vi "RMAD logger.vi"() -> ()   [LabVIEW 2017]
panel:
  out "regobs from inifile":T1(array[cluster]) {"regobs_ObsLocation" items=["Ikke gitt"=0, "Lauvjuvet"=66553, "Sandneslia"=66555, "Lauvjuvet Demo"=47721, "Sandneslia Demo"=47724, "Lauvjuvet Test"=62943, "Sandneslia Test"=62942, "F46 test"=63942, "F46 Demo"=47760]; "regobs_AvalancheTriggerTID" items=["Ikke gitt"=0, "Naturlig utløst"=10, "Kunstig utløst"=20, "Ski eller skuter utløst"=21, "Ski eller skuter fjernutløst"=22, "Kunstig utløst testheng"=23, "Utløst med sprengstoff"=25, "Ukjent"=99]; "regobs_AvalancheTID" items=["Ikke gitt"=0, "Tørt løssnøskred"=12, "Vått løssnøskred"=11, "Tørt flakskred"=22, "Vått flakskred"=21, "Glideskred"=27, "Sørpeskred"=30, "Skavlfall"=40, "Ukjent"=99]; "regobs_TerrainStartZoneTID" items=["Ikke gitt"=0, "Brattheng"=10, "Leområder"=20, "Nær rygg"=30, "I renne eller forsenkning"=40, "Svaberg"=50, "Skål"=60, "I skogen"=70, "Hogstfelt"=75, "Overalt i terrenget"=95, "Ukjent"=99]}
  out "Trafikkontroll terskelverdier":T2(array[cluster])
  out "Stredstørrelser terskelverdier":T3(array[cluster])
  in  "Tab Control":T4(tab)
  out "Skredhendelser":T5(array[cluster]) {"Intensitet terskel 1" format="%.1f"; "Intensitet terskel 2" format="%.1f"; "Intensitet terskel 3" format="%.1f"; "Intensitet terskel 4" format="%.1f"; "Intensitet terskel 5" format="%.1f"}
  out "is logging":bool[](array[boolean])
  out "registration in regObs":T6(array[cluster]) {"DestructiveSizeTID" items=["Ikke gitt"=0, "1-Harmløs"=1, "2-Små"=2, "3-Middels"=3, "4-Stort"=4, "5-Svært stort"=5, "Ukjent"=9]; "TerrainStartZoneTID" items=["Ikke gitt"=0, "Brattheng"=10, "Leområder"=20, "Nær rygg"=30, "I renne eller forsenkning"=40, "Svaberg"=50, "Skål"=60, "I skogen"=70, "Hogstfelt"=75, "Overalt i terrenget"=95, "Ukjent"=99]; "AvalancheTID" items=["Ikke gitt"=0, "Tørt løssnøskred"=12, "Vått løssnøskred"=11, "Tørt flakskred"=22, "Vått flakskred"=21, "Glideskred"=27, "Sørpeskred"=30, "Skavlfall"=40, "Ukjent"=99]; "AvalancheTriggerTID" items=["Ikke gitt"=0, "Naturlig utløst"=10, "Kunstig utløst"=20, "Ski eller skuter utløst"=21, "Ski eller skuter fjernutløst"=22, "Kunstig utløst testheng"=23, "Utløst med sprengstoff"=25, "Ukjent"=99]}
  out "registration ID":string[](array[string])
  in  "?":T7(tab)
  out "Nedlastede data 1":waveform(dbl)[](graph)
  out "Nedlastede data 2":waveform(dbl)[](graph)
  out "Nedlastede data 3":waveform(dbl)[](graph)
  out "Nedlastede data 4":waveform(dbl)[](graph)
  out "Nedlastede data 5":waveform(dbl)[](graph)
  in  "Download dataset":bool
  in  "Node":i32=1
  in  "ID":u16
  in  "Start Logging":bool
  out "Recent events":T8(array[cluster]) {"SPS" format="%.1f"}
  out "Temperatur":waveform(dbl)[](graph)
  out "Batteri spenning":waveform(dbl)[](graph)
  out "Radio Latency":waveform(i32)[](graph)
  out "Avalanch Packets":T9(array[cluster]) {"A1 std" format="%.1f"; "A2 std" format="%.1f"; "A3 std" format="%.1f"; "A4 std" format="%.1f"; "A1 ratio" format="%.1g"; "A2 ratio" format="%.1g"; "A3 ratio" format="%.1g"; "A4 ratio" format="%.1g"}
  out "Avalanch JBV":T10(array[cluster]) {"A2 mean" format="%.1f"; "A1 mean" format="%.1f"; "A1 std" format="%.1f"; "A2 std" format="%.1f"}
  in  "Send Reset":bool
  in  "SetAUX":bool
  in  "Node":u8=1
  in  "Get Status":bool
  in  "AUX min int":u16=15
  out "AUX data":T11(array[cluster]) {"Node configuration"."configuration" items=[""=100, "Radio Repeater"=0, "Geofon"=1, "Sensornode"=2, "Jernbane"=3, "Infralyd"=4]; "Node configuration"."radio config" items=[""=100, "Smartmesh IP"=0]; "batteri (V)" format="%.3g"; "temperatur (c)" format="%.1g"; "?" format="%#.5g"}
  out "Mote Status":T12(array[cluster]) {"mote state" items=["Lost"=0, "Negotiating"=1, "Operational"=4]}
  out "Link status":T13(array[cluster])
  out "Safe download":T14(array[cluster])
  out "NGI Packets Dust":cluster{"MAc Adress":string, "data":string}[](array[cluster])
  out "dust manager mac adress":string
  out "mac adress":string[](array[string])
  out "radio IO":errorcluster
  in  "stop":bool
  out "gateway IP":T15={"serial_mux IP"="127.0.0.1", "serial_mux port"=9900}
  out "event_datadir":string
  out "aux_datadir":string
  out "mesh_datadir":string
  out "sec since last packet":dbl
  out "Gateway Info":T16
  out "Gateway Status":T17
  out "node names":string[](array[string])
  in  "max download atempts":u8=3
  out "auto_download_enabled":bool
  out "gateway_snmp_enabled":bool
  out "RMAD signalys monitor enabled":bool
  out "vdv_datadir":string
  out "ini file":path
  out "regObs baseurl":string
  out "RMAD Signalys Monitor":T18 {"Uptime  (W:D:H)" format="%<%W:%D:%H>t"}
  out "error regObs":errorcluster
  out "error signalys":errorcluster
  out "error snmp":errorcluster
  in  "download timeout":dbl=180.0 format="%#_13g"
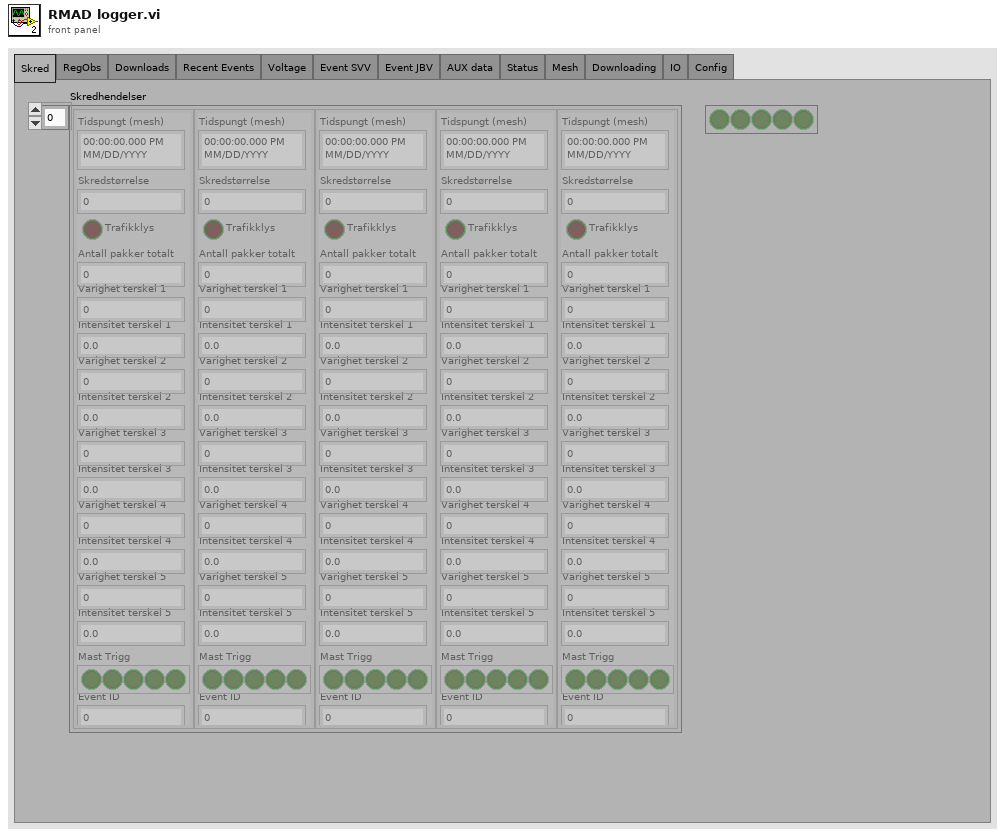
[diagram p1: front panel]
types:
  T1 = cluster{"regobs_ObsLocation":i32, "regobs_AvalancheTriggerTID":i32, "regobs_AvalancheTID":i32, "regobs_TerrainStartZoneTID":i32, "regobs_Trajectory":string, "regobs_ValidExposition":string, "regobs_startLat":dbl, "regobs_startLong":dbl, "regobs_stopLat":dbl[], "regobs_stopLong":dbl[], "regobs_heading":u32, "regobs_velocity":u32, "regobs_comment":string}[]
  T2 = cluster{"terskelverdi":u32, "antall sensorer":u32, "varighet":u32}[]
  T3 = cluster{"teskelverdi":u32, "antall sensorer":u32, "varighet":u32}[][]
  T4 = enum32{"Skred", "RegObs", "Downloads", "Recent Events", "Voltage", "Event SVV", "Event JBV", "AUX data", "Status", "Mesh", "Downloading", "IO", "Config"}
  T5 = cluster{"Tidspungt (mesh)":timestamp, "Skredstørrelse":i32, "Trafikklys":bool, "Antall pakker totalt":u16, "Varighet terskel 1":u16, "Intensitet terskel 1":dbl, "Varighet terskel 2":u16, "Intensitet terskel 2":dbl, "Varighet terskel 3":u16, "Intensitet terskel 3":dbl, "Varighet terskel 4":u16, "Intensitet terskel 4":dbl, "Varighet terskel 5":u16, "Intensitet terskel 5":dbl, "Mast Trigg":bool[], "Event ID":i32}[]
  T6 = cluster{"DtAvalancheTime (UTC)":string, "DestructiveSizeTID":i32, "AvalancheTriggerTID":i32, "AvalancheTID":i32, "TerrainStartZoneTID":i32, "ValidExposition":string, "Trajectory":string, "StartLat":dbl, "StartLong":dbl, "StopLat":dbl, "StopLong":dbl, "Comment":string}[]
  T7 = enum32{"Mast 1", "Mast 2", "Mast 3", "Mast 4", "Mast 5"}
  T8 = cluster{"ID":u16, "Timestamp":timestamp, "Packets":u16, "SPS":dbl, "Samples":u16}[][]
  T9 = cluster{"time (mesh)":timestamp, "Limit reached flagg":bool[], "A1 std":sgl, "A2 std":sgl, "A3 std":sgl, "A4 std":sgl, "A1 ratio":sgl, "A2 ratio":sgl, "A3 ratio":sgl, "A4 ratio":sgl, "A1 max":u16, "A2 max":u16, "A3 max":u16, "A4 max":u16, "A1 min":u16, "A2 min":u16, "A3 min":u16, "A4 min":u16, "A1 maxS":u16, "A2 maxS":u16, "A3 maxS":u16, "A4 maxS":u16, "A1 minS":u16, "A2 minS":u16, "A3 minS":u16, "A4 minS":u16}[]
  T10 = cluster{"Dust Timestamp":timestamp, "Limit reached flagg":bool[], "A1 std":sgl, "A2 std":sgl, "A1 mean":sgl, "A2 mean":sgl, "A1 max":i32, "A2 max":i32, "A1 min":i32, "A2 min":i32, "A1 maxS":u16, "A2 maxS":u16, "A1 minS":u16, "A2 minS":u16}[]
  T11 = cluster{"Node configuration":cluster{"configuration":u8, "sw vertion":u8, "hw revition":u8, "radio config":u8}, "flaggs":bool[], "batteri (V)":dbl, "temperatur (c)":dbl, "is singed int?":bool[], dbl[], "last update (pc time)":timestamp}[]
  T12 = cluster{"mac adress":string, "mote state":u8, "temperature (C)":i8, "battery (mV)":u16, "avg latecy":u32, "requested bw":u32, "good neighbour":u8, "num neighbour":u8, "num lost packets":u8, "last update (pc)":timestamp}[]
  T13 = cluster{"source mac adress":string, cluster{"destination":string, "rssi":i8, "TxPackets":u16}[], "last update":timestamp}[]
  T14 = cluster{"this instance":bool, "download ID":u32, "samples in dataset":u32, "num  samples":u32, "downloading":bool, "complete":bool, "attempts":u32, "timeout clock":timestamp}[]
  T15 = cluster{"serial_mux IP":string, "serial_mux port":u16}
  T16 = cluster{"Name":string, "Location":string, "Gateway":string, "Firmware":string, "Serial Number":string}
  T17 = cluster{"Supply Voltage":dbl, "Temperatur":u32, "DI":bool, "DO":bool}
  T18 = cluster{"Uptime  (W:D:H)":dbl, "status error":bool, "output enabled":bool, "Last update":timestamp}
  T19 = enum16{"big-endian, network order", "native, host order", "little-endian"}
  T20 = cluster{"Device Health Report":cluster{"MAC adress":string, "charge (mC)":u32, "queueOcc":u8, "temperature (C)":i8, "batteryVoltage (mV)":u16, "numTxOk":u16, "numTxFail":u16, "numRxOK":u16, "numRxFail":u16, "numMACdropped":u8, "numTxBad":u8, "badLinkFrameID":u8, "badLinkSlot":u32, "badLinkOffset":u8}, "mote staus event":cluster{"data":string, u8}, "getMoteInfo":cluster{"MAC adress":string, "state":u8, "numNbrs":u8, "numGoodNbrs":u8, "requestedBw":u32, "totalNeededBw":u32, "assignedBw":u32, "packetsRecived":u32, "packetsLost":u32, "avgLatecy":u32}, "GetPathInfo":cluster{"Path ID":u8, "Src MAC":string, "Dest MAC":string, "direction":u8, "numLinks":u8, "quality":u8, "rssiScrDest":i8, "rssiDestScr":i8}, "Neighbors Health Report":cluster{"MAC adress":string, "neighbourHRdata":cluster{"neighbourID":u16, "neighborFlag":u8, "rssi":i8, "numTxPackets":u16, "numTxFailures":u16, "numRxPackets":u16}[]}, "Discovered Nighbors Health Report":cluster{"MAC adress":string, "numJoinParents":u8, cluster{"neighborID":u16, "rssi":i8, "numRx":u8}[]}, "Mote Config":cluster{"mac adress":string, "MoteID":u16, "isAP":bool, "mote state":u8, "reserved":u8, "isRouting":bool}}
  T21 = cluster{"MAc Adress":string, "UTC Time":timestamp, "srcPort":u16, "dstPort":u16, "data":string}
  T22 = cluster{"Is logging":bool, "num avalanch":u16, "logging startet":timestamp}[]
  T23 = cluster{"ID":u16, "CH mask":u8, "First scan":u32, "Last scans":u32, "Samples":i32[][]}[]
  T24 = cluster{"Dust Timestamp":timestamp, "Limit reached flagg":bool[], "A1 std":sgl, "A2 std":sgl, "A3 std":sgl, "A4 std":sgl, "A1 rat":sgl, "A2 rat":sgl, "A3 rat":sgl, "A4 rat":sgl, "A1 max":u16, "A2 max":u16, "A3 max":u16, "A4 max":u16, "A1 min":u16, "A2 min":u16, "A3 min":u16, "A4 min":u16, "A1 maxS":u16, "A2 maxS":u16, "A3 maxS":u16, "A4 maxS":u16, "A1 minS":u16, "A2 minS":u16, "A3 minS":u16, "A4 minS":u16}[]
  T25 = cluster{"Tidspungt (mesh)":timestamp, "Skredstørrelse":u16, "Trafikklys":bool, "Antall pakker totalt":u16, "Varighet terskel 1":u16, "Intensitet terskel 1":dbl, "Varighet terskel 2":u16, "Intensitet terskel 2":dbl, "Varighet terskel 3":u16, "Intensitet terskel 3":dbl, "Varighet terskel 4":u16, "Intensitet terskel 4":dbl, "Varighet terskel 5":u16, "Intensitet terskel 5":dbl, "Mast Trigg":bool[], "Event ID":i32}[]
  T26 = cluster{"DtAvalancheTime":string, "DestructiveSizeTID":i32, "AvalancheTriggerTID":i32, "AvalancheTID":i32, "TerrainStartZoneTID":i32, "ValidExposition":string, "Trajectory":string, "StartLat":dbl, "StartLong":dbl, "StopLat":dbl, "StopLong":dbl, "Comment":string}[]
  T27 = cluster{"this instance":bool, "download ID":u32, "samples in dataset":u32, "num downloaded samples":u32, "is downloading":bool, "dataset complete":bool, "download attempts":u32, "timeout clock":timestamp}[]
  T28 = cluster{"Mote Temperature":waveform(i32)[], "Mote Battery":waveform(i32)[], "Mote Average Latency":waveform(i32)[]}
  T29 = cluster{"source mac adress":string, cluster{"destination mac":string, "rssi":i8, "numTxPackets":u16}[], "last update":timestamp}[]
  T30 = typedef "LVDateTimeRec.ctl" = cluster{"fractional second":dbl, "second":i32, "minute":i32, "hour":i32, "day of month":i32, "month":i32, "year":i32, "day of week":i32, "day of year":i32, "DST":i32}
  T31 = cluster{"serial_mux IP":string, "rserial_mux port":u16}
  T32 = cluster{"dust master mac":string, "xbee master mac":string, "master name":string, "dust mac":string[], "xbee mac":string[], "node names":string[]}
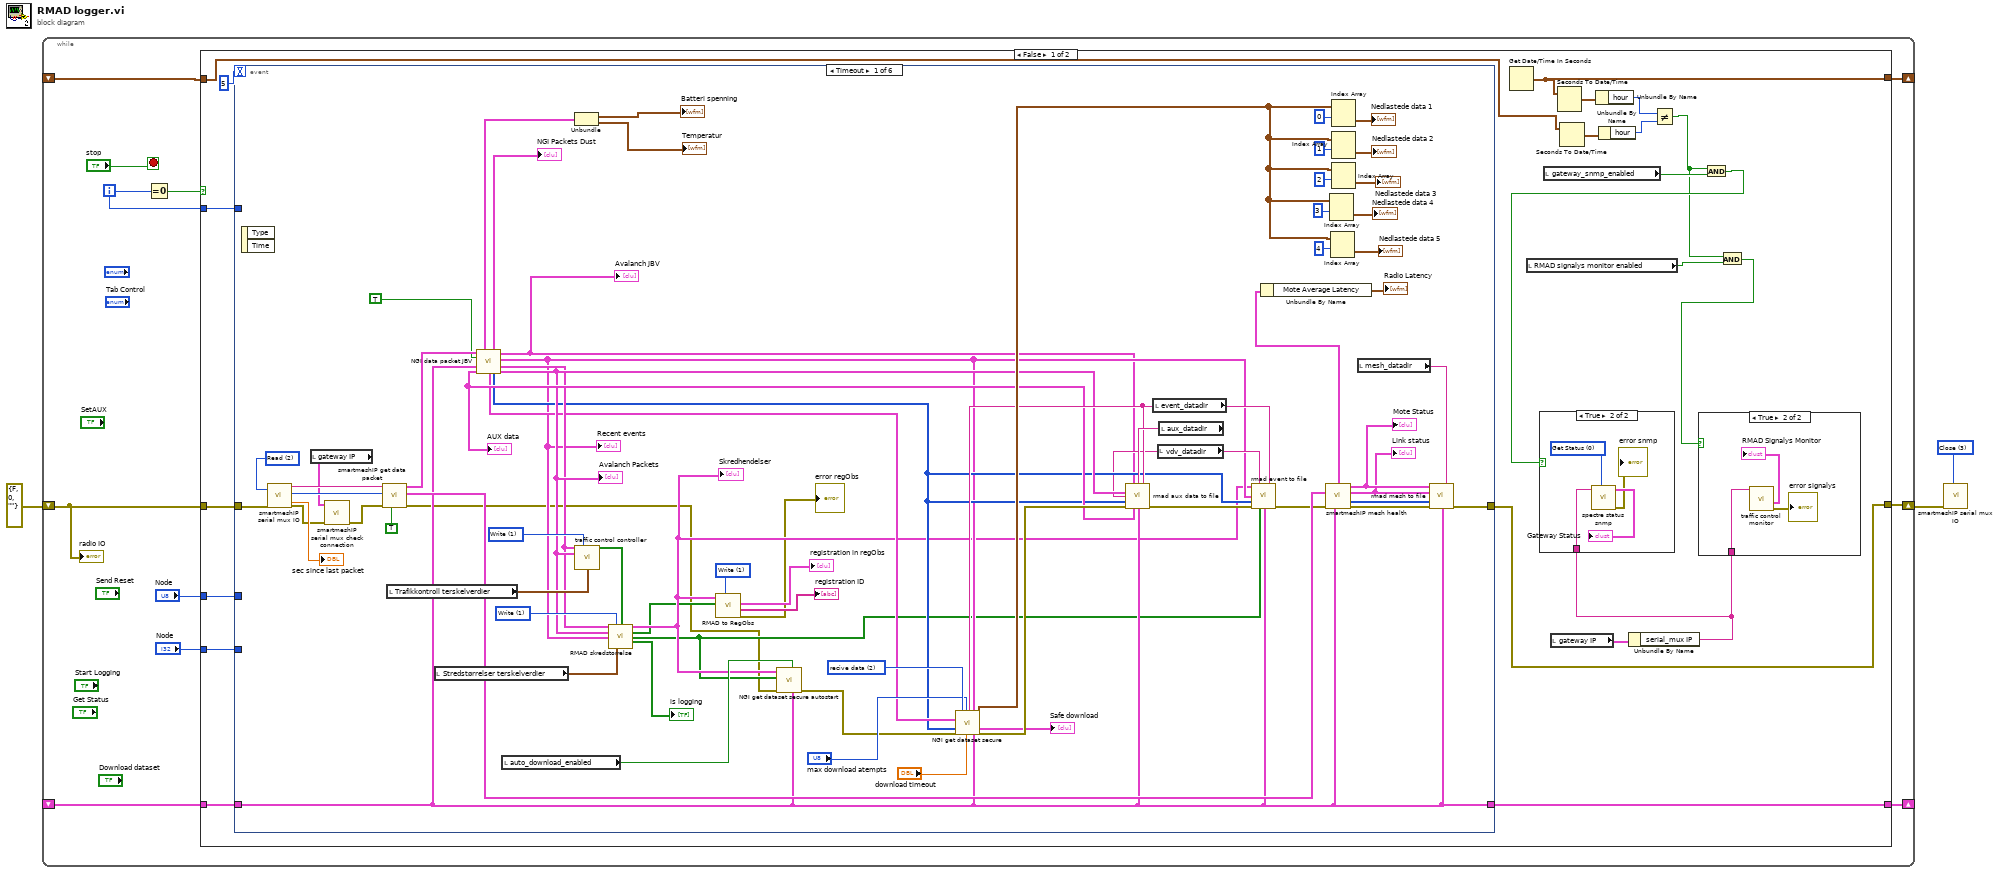
[diagram p0: block diagram]
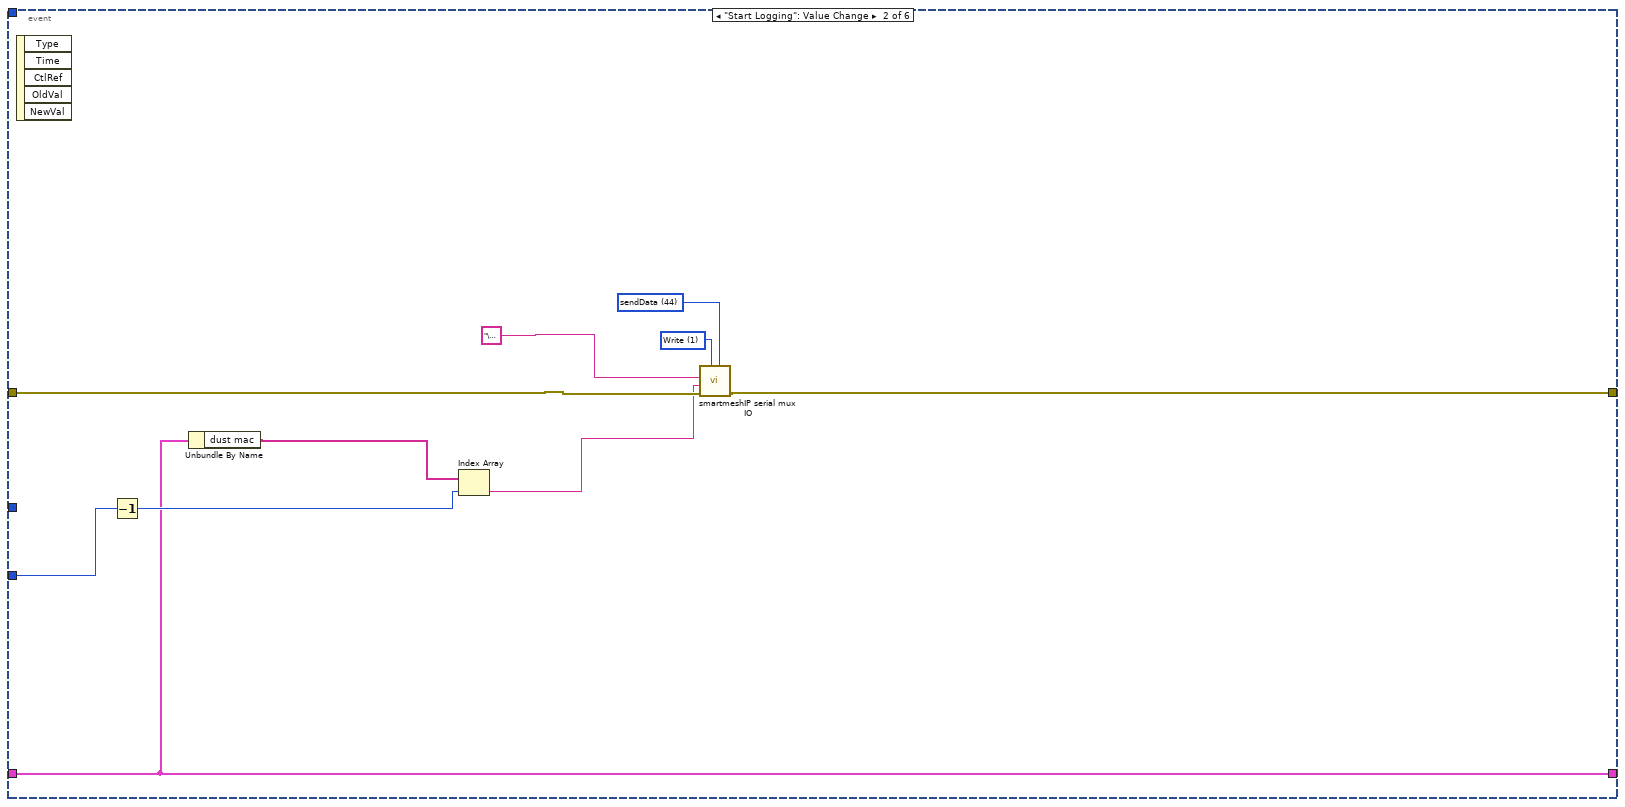
[diagram p4: hidden frame]
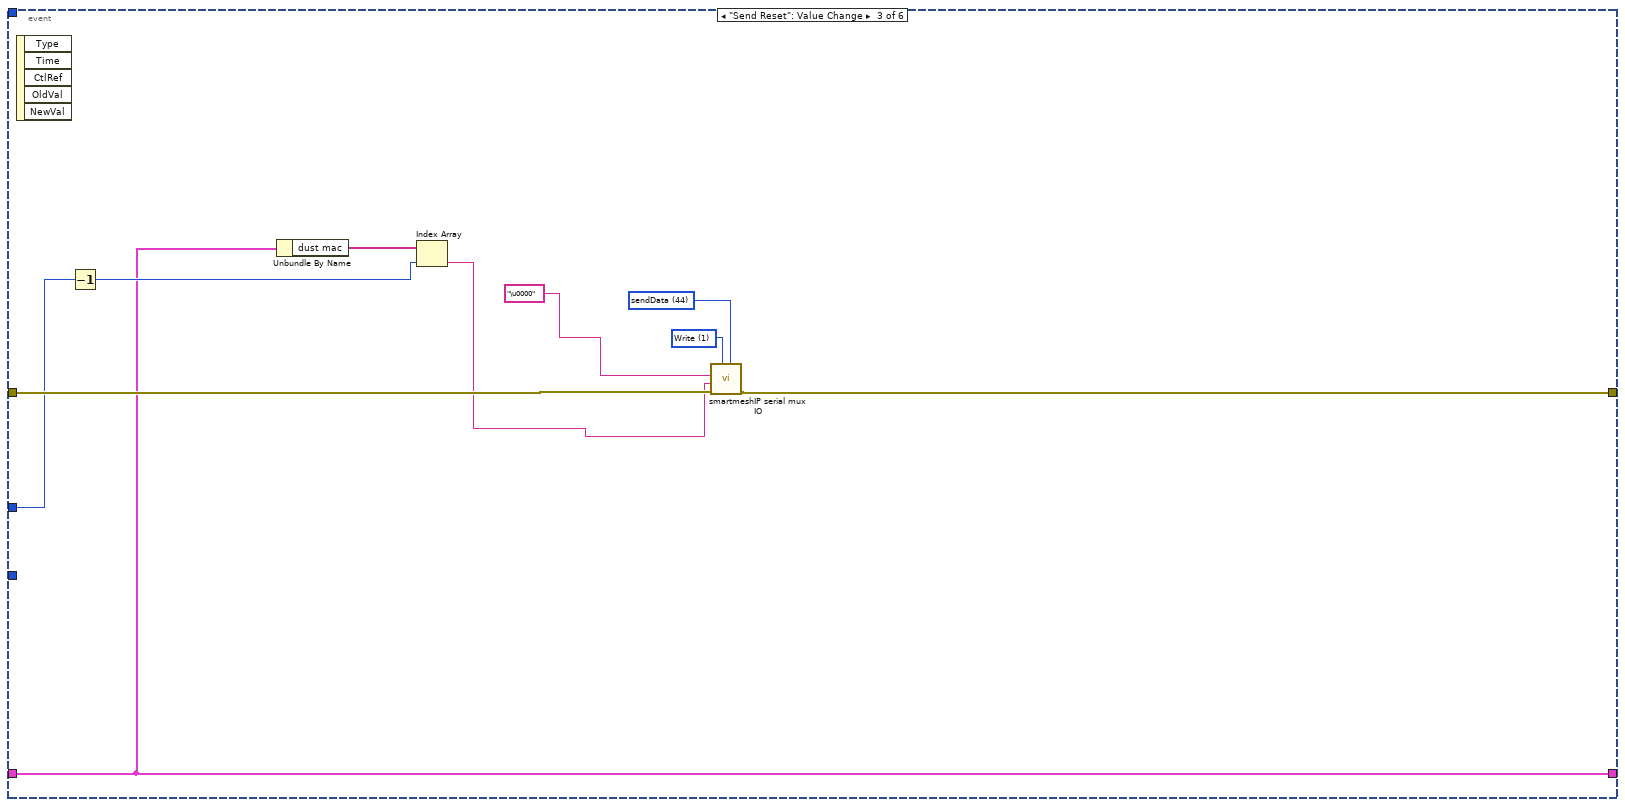
[diagram p5: hidden frame]
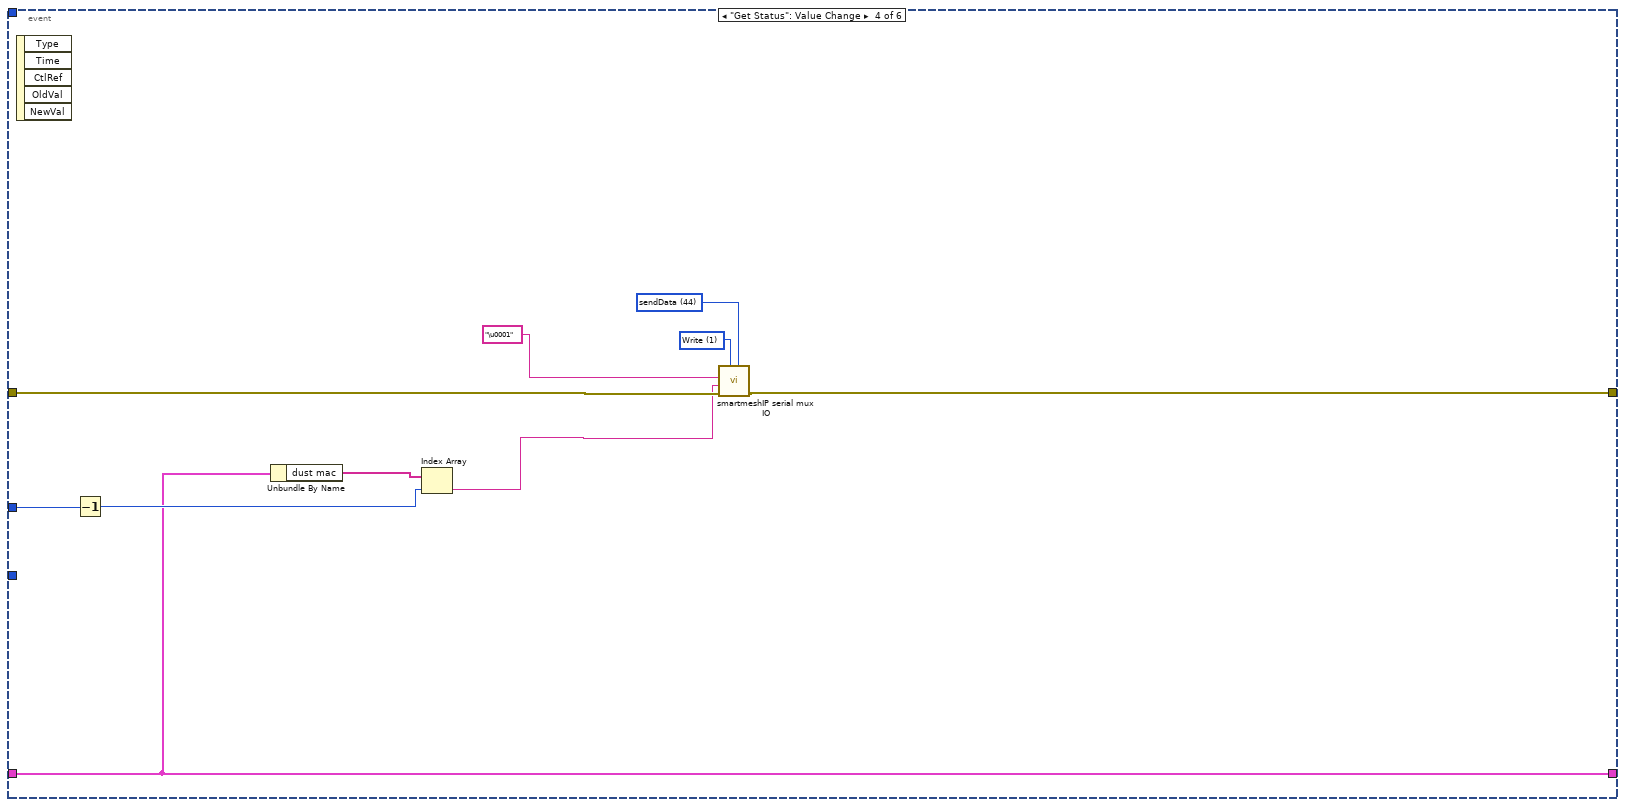
[diagram p6: hidden frame]
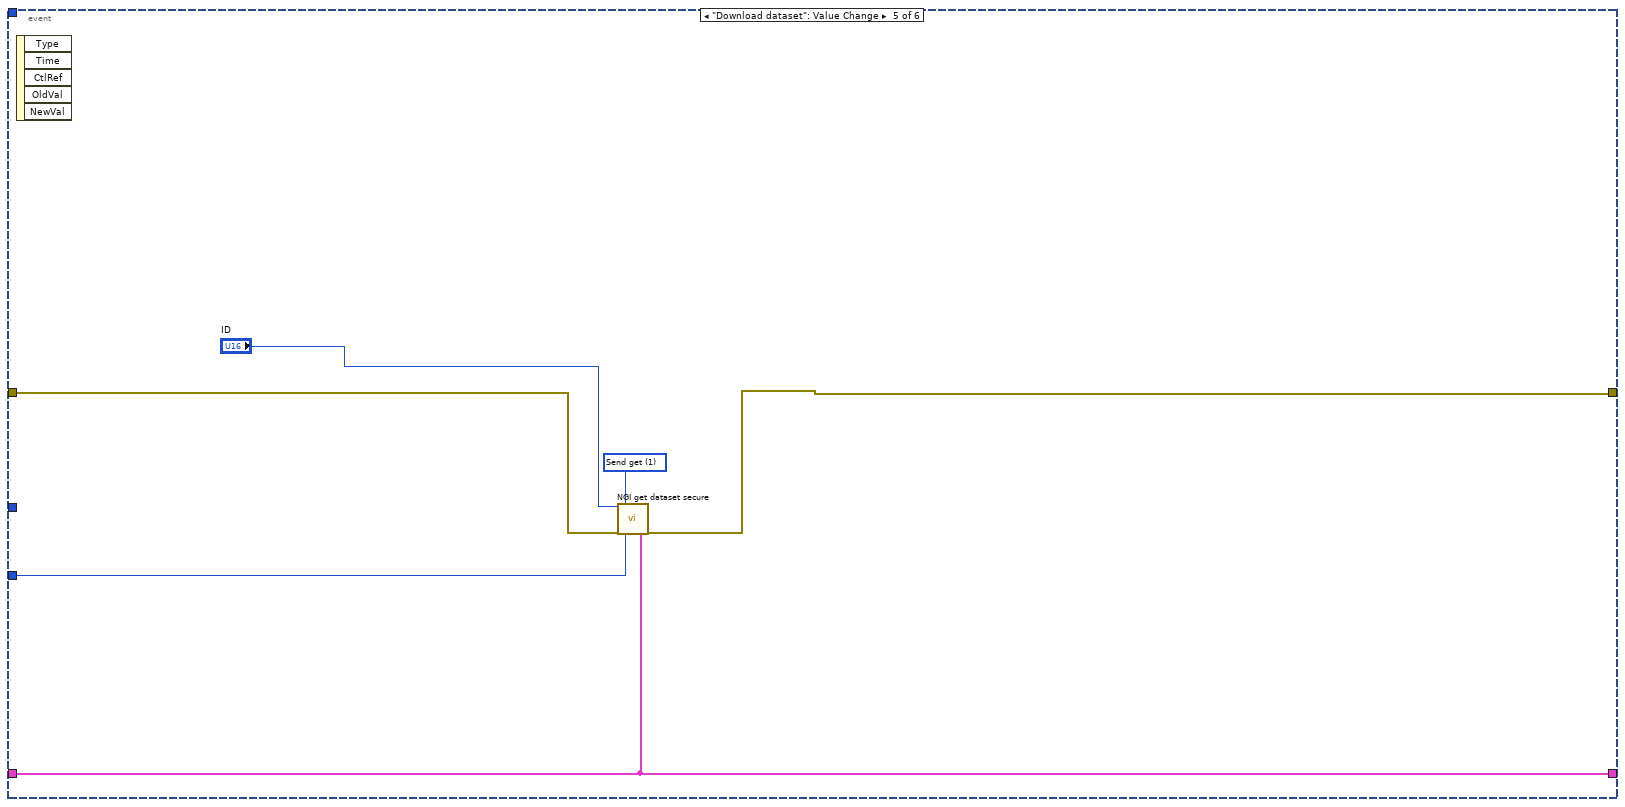
[diagram p7: hidden frame]
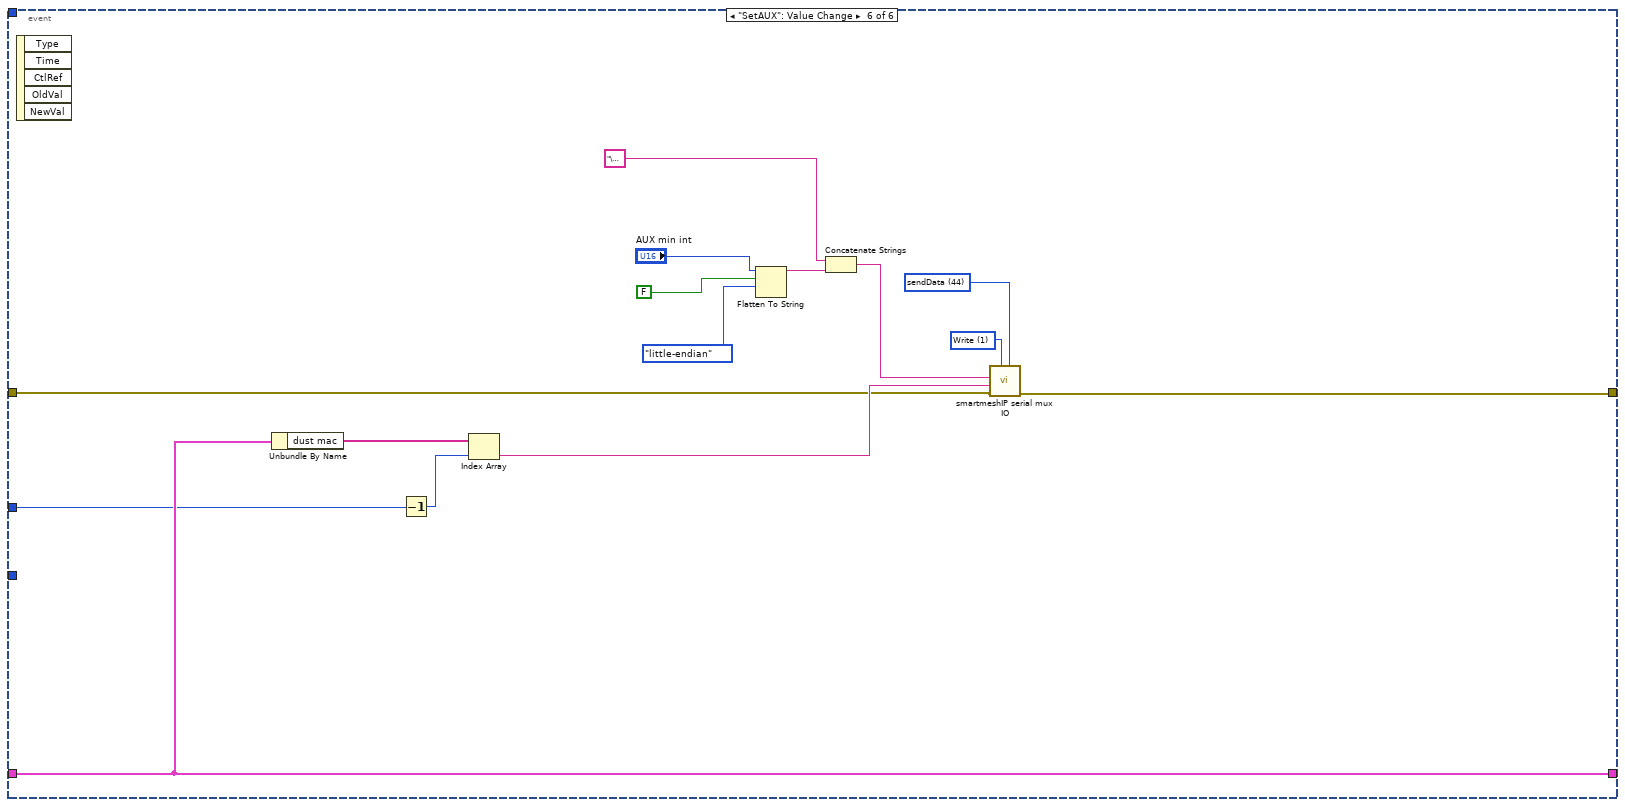
[diagram p8: hidden frame]
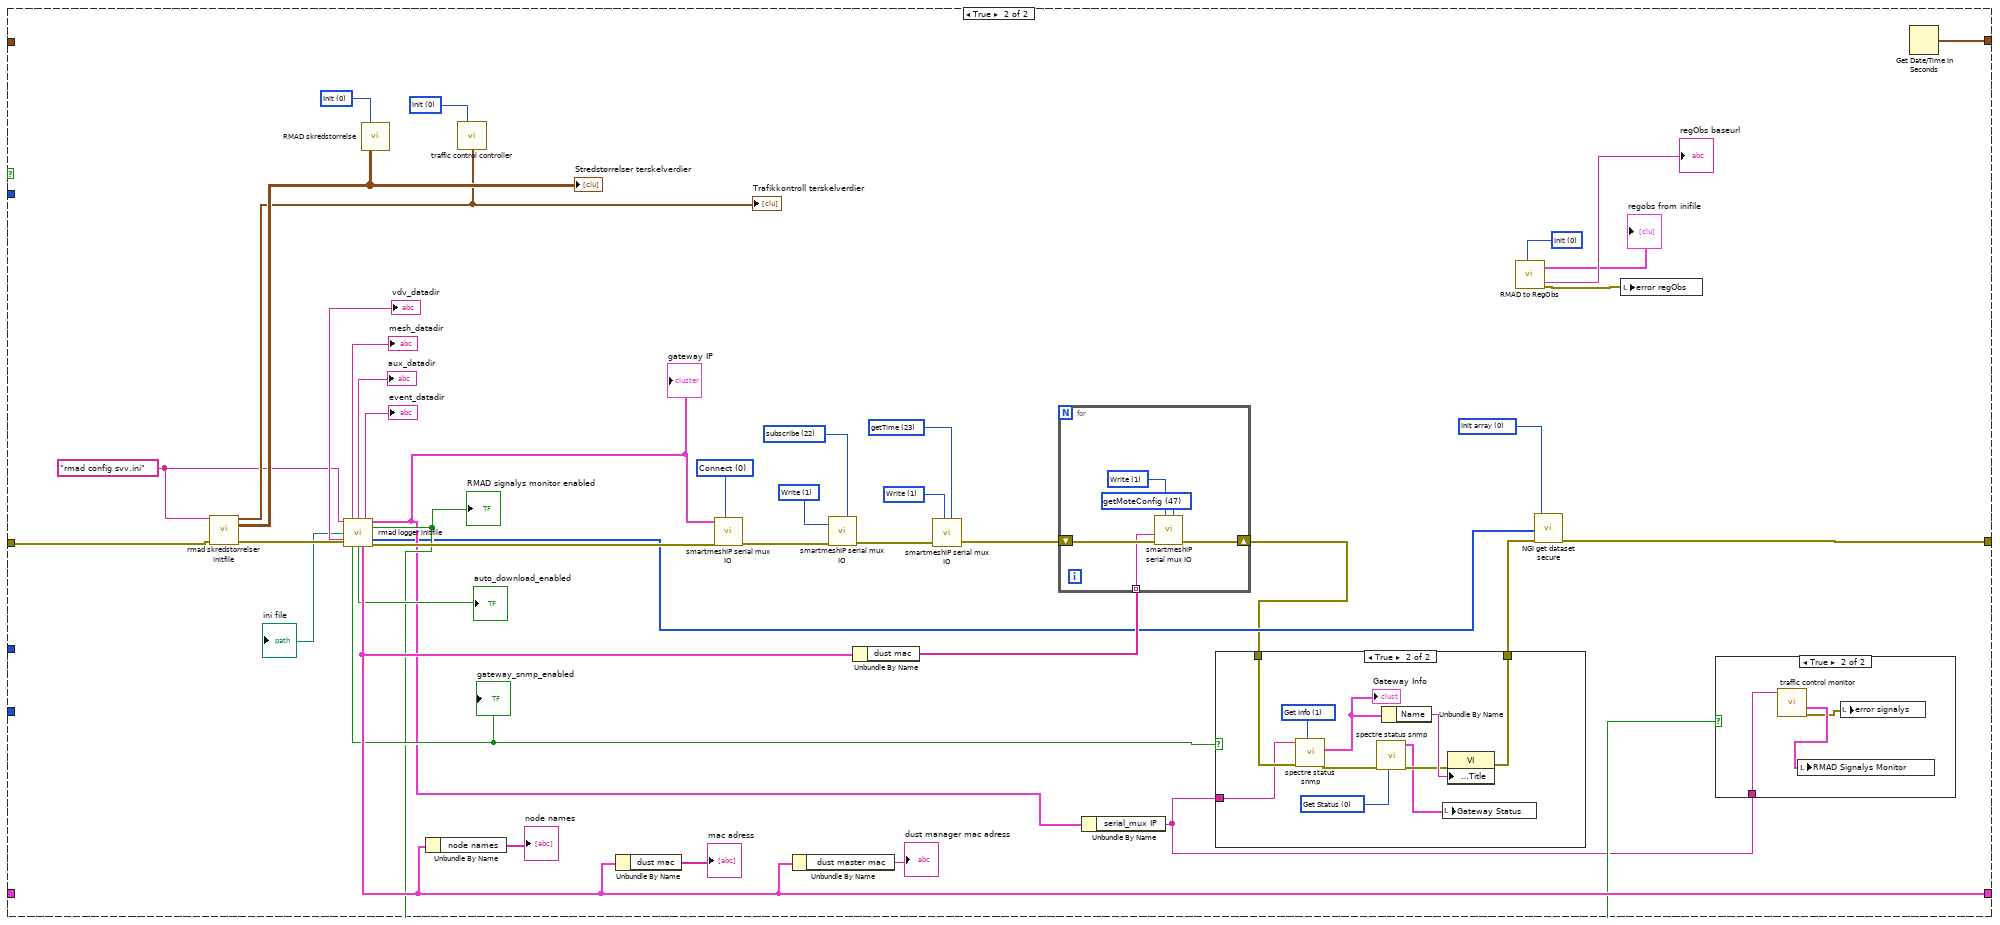
[diagram p9: hidden frame]
diagram:
  w3 = u16 3 items=["Connect", "Write", "Read", "Close"] ("State")
  n1 = while {
    shift-right: [w13] -> w2
    shift-left: errorcluster {"status"=FALSE, "code"=0, "source"=""} ("error out") -> [w7]
    shift-right: [w9] -> _
    shift-left: _ -> [w8]
    shift-right: [w5] -> _
    shift-left: _ -> [w4]
    i -> [w6]
    stop <- "stop" stop-if-true
    n2 = Equal To 0?(x=w6) -> (x = 0?=w14:bool)
    n3 = case shown="False" w14 {
      tunnel: [w15 w163] -> w13
      tunnel: w7 -> [w35 w179]
      tunnel: w6 -> [w33 _]
      tunnel: "Node" -> [w32 _]
      tunnel: "Node" -> [w31 _]
      tunnel: [w24 w185] -> w9
      tunnel: w8 -> [w30 _]
      tunnel: [w29 w187] -> w5
      tunnel: w4 -> [w22 _]
      frame False {
        n4 = event shown="[0] Timeout" {
          selector: _ -> [_ _ _ _ _ _]
          dyn-events: _ -> [_ _ _ _ _ _]
          timeout: 5 -> [_ _ _ _ _ _]
          tunnel: w35 -> [w111 w117 w128 w137 w146 w157]
          tunnel: [w53 w115 w127 w134 w142 w153] -> w15
          tunnel: w33 -> [_ _ _ _ _ _]
          tunnel: w32 -> [_ _ w122 w141 _ w150]
          tunnel: w31 -> [_ w120 _ _ w147 _]
          tunnel: w30 -> [w65 w112 w125 w133 w143 w155]
          tunnel: [w65 w112 w125 w133 w143 w155] -> w24
          event Timeout {
            w57 = u16 1 items=["Init", "Write"] ("State")
            w78 = u16 1 items=["Init", "Write"] ("State")
            w83 = u16 2 items=["Init array", "Send get", "recive data", "Close"] ("State")
            w94 = u16 1 items=["Init", "Write"] ("State")
            w110 = u16 2 items=["Connect", "Write", "Read", "Close"] ("State")
            n5 = event-data() -> ()  [unwired: 1 in, 2 out]
            n6 = call "smartmeshIP serial mux IO.vi"("State"=w110, "error in"=w111) -> ("error out"=w52:errorcluster, "rx_commandType"=w101:u8, "rx_data"=w102:string, "sec since last packet"=→"sec since last packet":dbl)  [unwired: 4 in, 2 out]
            n7 = local read "gateway IP"() -> (w95:T15)
            n8 = call "smartmeshIP serial mux check connection.vi"("error in"=w52, "serial mux adress"=w95) -> ("error out"=w87:errorcluster)  [unwired: 8 in, 1 out]
            n9 = call "smartmeshIP get data packet.vi"("use correction"=TRUE ("use time correction"), "error in"=w87, "commandType"=w101, "data"=w102) -> ("error out"=w46:errorcluster, "mote and link status"=w100:T20, "Data Notifications"=w66:T21)  [unwired: 5 in]
            n10 = local read "Trafikkontroll terskelverdier"() -> (w72:T2)
            n11 = local read "Stredstørrelser terskelverdier"() -> (w73:T3)
            n12 = call "NGI data packet JBV.vi"("Dust Data Notifications"=w66, "list only event > 0"=TRUE, "mac adresses"=w65) -> ("output waveforms"=w67:cluster{waveform(dbl)[], waveform(dbl)[]}, "NGI  packets dust"=→"NGI Packets Dust":cluster{"MAc Adress":string, "data":string}[], "Avalanch JBV"=w43:T10, "Recent events"=w58:T8, "Is Logging"=w62:T22, "AUX data"=w64:T11, "Downloaded dataset"=w61:T23, "last packet type"=w60:u8[], "Avalanch Packets"=w63:T24)  [unwired: 3 in, 1 out]
            "Avalanch Packets" <- w63
            "AUX data" <- w64
            "Recent events" <- w58
            "Avalanch JBV" <- w43
            n13 = local read "auto_download_enabled"() -> (w68:bool)
            n14 = Unbundle(w67) -> (→"Batteri spenning":waveform(dbl)[], →"Temperatur":waveform(dbl)[])
            n15 = call "traffic control controller.vi"("Is Logging"=w62, "State"=w94, "Avalanch Packets"=w63, "Trafikkontroll terskelverdier"=w72) -> ("Rød mast"=w71:bool[])  [unwired: 9 in, 2 out]
            n16 = call "RMAD skredstorrelse.vi"("Is Logging"=w62, "State"=w78, "Rød signal kriterie"=w71, "Avalanch Packets"=w63, "Recent events"=w58, "Stredstørrelser terskelverdier"=w73) -> ("Skredhendelser"=w56:T25, "event to regobs"=w47:bool[], "event to file?"=w48:bool[], "is logging"=→"is logging":bool[])  [unwired: 5 in, 1 out]
            "Skredhendelser" <- w56
            n17 = call "RMAD to RegObs.vi"("State"=w57, "skredhendelse to regobs?"=w47, "Skredhendelser"=w56) -> ("error out"=→"error regObs":errorcluster, "registration ID"=→"registration ID":string[], "registration in regObs"=→"registration in regObs":T26)  [unwired: 3 in, 3 out]
            n18 = call "NGI get dataset secure autostart.vi"("mac adresses"=w65, "Auto download"=w68, "error in (no error)"=w46, "event to file?"=w48, "Skredhendelser"=w56) -> ("error out"=w49:errorcluster)  [unwired: 6 in]
            n19 = local read "event_datadir"() -> (w69:string)
            n20 = call "NGI get dataset secure.vi"("Downloaded dataset"=w61, "last packet type"=w60, "error in (no error)"=w49, "State"=w83, "max download atempts"="max download atempts", "download timeout"="download timeout", "event_datadir"=w69, "Recent events 2"=w58, "mac adresses"=w65) -> ("Dataset"=w82:waveform(dbl)[][], "Safe Download"=→"Safe download":T27, "error out"=w84:errorcluster)  [unwired: 7 in, 1 out]
            n21 = local read "vdv_datadir"() -> (w59:string)
            n22 = local read "aux_datadir"() -> (w74:string)
            n23 = call "rmad aux data to file.vi"("Avalanch JBV"=w43, "aux_datadir"=w74, "event_datadir"=w69, "Avalanch Packets"=w63, "vdv_datadir"=w59, "last packet type"=w60, "error in"=w84, "AUX data"=w64, "mac adresses"=w65) -> ("error out"=w76:errorcluster)  [unwired: 6 in]
            n24 = call "rmad event to file.vi"("Skredhendelser"=w56, "vdv_datadir"=w59, "event_datadir"=w69, "Recent events 2"=w58, "last packet type"=w60, "error in"=w76, "event to file?"=w48, "mac adresses"=w65) -> ("error out"=w75:errorcluster)  [unwired: 7 in]
            n25 = call "smartmeshIP mesh health.vi"("mote and link status"=w100, "error in"=w75, "mac adresses"=w65) -> ("waveform output cluster"=w80:T28, "Mote Status"=w99:T12, "Primary link status"=w98:T29, "last packet type dust"=w86:i32[], "error out"=w81:errorcluster)  [unwired: 7 in, 1 out]
            "Mote Status" <- w99
            "Link status" <- w98
            n26 = Unbundle By Name(w80) -> ("Mote Average Latency"=→"Radio Latency":waveform(i32)[])
            n27 = Index Array(array=w82, index (row)=3) -> (element=→"Nedlastede data 4":waveform(dbl)[])  [unwired: 1 in]
            n28 = Index Array(array=w82, index (row)=4) -> (element=→"Nedlastede data 5":waveform(dbl)[])  [unwired: 1 in]
            n29 = Index Array(array=w82, index (row)=0) -> (element=→"Nedlastede data 1":waveform(dbl)[])  [unwired: 1 in]
            n30 = Index Array(array=w82, index (row)=1) -> (element=→"Nedlastede data 2":waveform(dbl)[])  [unwired: 1 in]
            n31 = Index Array(array=w82, index (row)=2) -> (element=→"Nedlastede data 3":waveform(dbl)[])  [unwired: 1 in]
            n32 = local read "mesh_datadir"() -> (w93:string)
            n33 = call "rmad mesh to file.vi"("Mote Status"=w99, "mesh datadir"=w93, "Primary link status"=w98, "last packet type dust"=w86, "error in"=w81, "mac adresses"=w65) -> ("error out"=w53:errorcluster)  [unwired: 9 in]
          }
          event "Start Logging": Value Change {
            w119 = u8 44 items=["subscribe"=22, "startNetwork"=45, "setUser"=58, "setTime"=54, "setNetworkConfig"=26, "setLicense"=56, "setIPConfig"=68, "setDownstreamFrameMode"=51, "setCommonJoinKey"=66, "setAdvertising"=50, "setACLEntry"=39, "sendIP"=59, "sendData"=44, "restorFactoryDefaults"=61, "reset"=21, "radiotestTx"=35, "radiotestRx"=37, "pingMote"=42, "getTime"=23, "getSystemInfo"=46, "radiotestStatistics"=38, "getPathInfo"=48, "getNextPath"=49, "getNextACLEntry"=40, "getNetworkInfo"=64, "getNetworkConfig"=63, "getMoteLinks"=70, "getMoteInfo"=62, "getMoteConfigByld"=65, "getMoteConfig"=47, "getManagerStatistics"=53, "getLog"=43, "getLicense"=55, "getIPConfig"=67, "exchangeNetworkID"=34, "exchangeMoteJoinKey"=33, "deleteMote"=69, "deleteACLEntry"=41, "clearStatistics"=31] ("commandType_write")
            w118 = u16 1 items=["Connect", "Write", "Read", "Close"] ("State")
            n34 = event-data() -> ()  [unwired: 1 in, 5 out]
            n35 = Decrement(x=w120) -> (x-1=w121:i32)
            n36 = Unbundle By Name(w112) -> ("dust mac"=w113:string[])
            n37 = Index Array(array=w113, index=w121) -> (element=w114:string)
            n38 = call "smartmeshIP serial mux IO.vi"("tx_commandType"=w119, "State"=w118, "error in"=w117, "MAC source"=w114, "tx_data"="\u0004") -> ("error out"=w115:errorcluster)  [unwired: 1 in, 5 out]
          }
          event "Send Reset": Value Change {
            w130 = u8 44 items=["subscribe"=22, "startNetwork"=45, "setUser"=58, "setTime"=54, "setNetworkConfig"=26, "setLicense"=56, "setIPConfig"=68, "setDownstreamFrameMode"=51, "setCommonJoinKey"=66, "setAdvertising"=50, "setACLEntry"=39, "sendIP"=59, "sendData"=44, "restorFactoryDefaults"=61, "reset"=21, "radiotestTx"=35, "radiotestRx"=37, "pingMote"=42, "getTime"=23, "getSystemInfo"=46, "radiotestStatistics"=38, "getPathInfo"=48, "getNextPath"=49, "getNextACLEntry"=40, "getNetworkInfo"=64, "getNetworkConfig"=63, "getMoteLinks"=70, "getMoteInfo"=62, "getMoteConfigByld"=65, "getMoteConfig"=47, "getManagerStatistics"=53, "getLog"=43, "getLicense"=55, "getIPConfig"=67, "exchangeNetworkID"=34, "exchangeMoteJoinKey"=33, "deleteMote"=69, "deleteACLEntry"=41, "clearStatistics"=31] ("commandType_write")
            w129 = u16 1 items=["Connect", "Write", "Read", "Close"] ("State")
            n39 = event-data() -> ()  [unwired: 1 in, 5 out]
            n40 = Decrement(x=w122) -> (x-1=w131:u8)
            n41 = Unbundle By Name(w125) -> ("dust mac"=w124:string[])
            n42 = Index Array(array=w124, index=w131) -> (element=w126:string)
            n43 = call "smartmeshIP serial mux IO.vi"("tx_commandType"=w130, "State"=w129, "error in"=w128, "MAC source"=w126, "tx_data"="\u0000") -> ("error out"=w127:errorcluster)  [unwired: 1 in, 5 out]
          }
          event "Get Status": Value Change {
            w139 = u8 44 items=["subscribe"=22, "startNetwork"=45, "setUser"=58, "setTime"=54, "setNetworkConfig"=26, "setLicense"=56, "setIPConfig"=68, "setDownstreamFrameMode"=51, "setCommonJoinKey"=66, "setAdvertising"=50, "setACLEntry"=39, "sendIP"=59, "sendData"=44, "restorFactoryDefaults"=61, "reset"=21, "radiotestTx"=35, "radiotestRx"=37, "pingMote"=42, "getTime"=23, "getSystemInfo"=46, "radiotestStatistics"=38, "getPathInfo"=48, "getNextPath"=49, "getNextACLEntry"=40, "getNetworkInfo"=64, "getNetworkConfig"=63, "getMoteLinks"=70, "getMoteInfo"=62, "getMoteConfigByld"=65, "getMoteConfig"=47, "getManagerStatistics"=53, "getLog"=43, "getLicense"=55, "getIPConfig"=67, "exchangeNetworkID"=34, "exchangeMoteJoinKey"=33, "deleteMote"=69, "deleteACLEntry"=41, "clearStatistics"=31] ("commandType_write")
            w138 = u16 1 items=["Connect", "Write", "Read", "Close"] ("State")
            n44 = event-data() -> ()  [unwired: 1 in, 5 out]
            n45 = Decrement(x=w141) -> (x-1=w140:u8)
            n46 = Unbundle By Name(w133) -> ("dust mac"=w132:string[])
            n47 = Index Array(array=w132, index=w140) -> (element=w135:string)
            n48 = call "smartmeshIP serial mux IO.vi"("tx_commandType"=w139, "State"=w138, "error in"=w137, "MAC source"=w135, "tx_data"="\u0001") -> ("error out"=w134:errorcluster)  [unwired: 1 in, 5 out]
          }
          event "Download dataset": Value Change {
            w145 = u16 1 items=["Init array", "Send get", "recive data", "Close"] ("State")
            n49 = event-data() -> ()  [unwired: 1 in, 5 out]
            n50 = call "NGI get dataset secure.vi"("ID"="ID", "error in (no error)"=w146, "State"=w145, "Node"=w147, "mac adresses"=w143) -> ("error out"=w142:errorcluster)  [unwired: 11 in, 3 out]
          }
          event "SetAUX": Value Change {
            w160 = u8 44 items=["subscribe"=22, "startNetwork"=45, "setUser"=58, "setTime"=54, "setNetworkConfig"=26, "setLicense"=56, "setIPConfig"=68, "setDownstreamFrameMode"=51, "setCommonJoinKey"=66, "setAdvertising"=50, "setACLEntry"=39, "sendIP"=59, "sendData"=44, "restorFactoryDefaults"=61, "reset"=21, "radiotestTx"=35, "radiotestRx"=37, "pingMote"=42, "getTime"=23, "getSystemInfo"=46, "radiotestStatistics"=38, "getPathInfo"=48, "getNextPath"=49, "getNextACLEntry"=40, "getNetworkInfo"=64, "getNetworkConfig"=63, "getMoteLinks"=70, "getMoteInfo"=62, "getMoteConfigByld"=65, "getMoteConfig"=47, "getManagerStatistics"=53, "getLog"=43, "getLicense"=55, "getIPConfig"=67, "exchangeNetworkID"=34, "exchangeMoteJoinKey"=33, "deleteMote"=69, "deleteACLEntry"=41, "clearStatistics"=31] ("commandType_write")
            w159 = u16 1 items=["Connect", "Write", "Read", "Close"] ("State")
            n51 = event-data() -> ()  [unwired: 1 in, 5 out]
            n52 = Unbundle By Name(w155) -> ("dust mac"=w154:string[])
            n53 = Decrement(x=w150) -> (x-1=w156:u8)
            n54 = Index Array(array=w154, index=w156) -> (element=w158:string)
            n55 = Flatten To String(anything="AUX min int", prepend array or string size? (T)=FALSE, byte order (0:big-endian, network order)=T19."little-endian") -> (data string=w151:string)  [unwired: 1 in, 2 out]
            n56 = Concatenate Strings("\u000b", w151) -> (w148:string)
            n57 = call "smartmeshIP serial mux IO.vi"("tx_commandType"=w160, "State"=w159, "error in"=w157, "MAC source"=w158, "tx_data"=w148) -> ("error out"=w153:errorcluster)  [unwired: 1 in, 5 out]
          }
        }
        n58 = Get Date/Time In Seconds() -> (seconds since 1Jan1904=w29:timestamp)
        n59 = local read "RMAD signalys monitor enabled"() -> (w16:bool)
        n60 = local read "gateway_snmp_enabled"() -> (w21:bool)
        n61 = local read "gateway IP"() -> (w23:T15)
        n62 = Seconds To Date/Time(time stamp (now)=w29) -> (date time rec=w28:T30)  [unwired: 1 in]
        n63 = Seconds To Date/Time(time stamp (now)=w22) -> (date time rec=w27:T30)  [unwired: 1 in]
        n64 = Unbundle By Name(w28) -> ("hour"=w26:i32)
        n65 = Unbundle By Name(w27) -> ("hour"=w25:i32)
        n66 = Unbundle By Name(w23) -> ("serial_mux IP"=w19:string)
        n67 = Not Equal?(x=w26, y=w25) -> (x != y?=w18:bool)
        n68 = And(x=w18, y=w21) -> (x .and. y?=w20:bool)
        n69 = case shown="True" w20 {
          tunnel: w19 -> [_ w42]
          frame False {
          }
          frame True {
            w41 = u16 0 items=["Get Status", "Get Info", "Get Uptime"] ("Ring")
            n70 = call "spectre status snmp .vi"("Ring"=w41, "IP Address"=w42) -> ("error out"=→"error snmp":errorcluster, "Gateway Status"=→"Gateway Status":T17)  [unwired: 6 in, 2 out]
          }
        }
        n71 = And(x=w18, y=w16) -> (x .and. y?=w17:bool)
        n72 = case shown="True" w17 {
          tunnel: w19 -> [_ w38]
          frame False {
          }
          frame True {
            n73 = call "traffic control monitor.vi"("address"=w38) -> ("error out"=→"error signalys":errorcluster, "RMAD Signalys Monitor"=→"RMAD Signalys Monitor":T18)  [unwired: 7 in, 2 out]
          }
        }
      }
      frame True {
        w169 = u16 0 items=["Init", "Write"] ("State")
        w171 = "rmad config svv.ini" ("initfile")
        w182 = u16 0 items=["Init", "Write"] ("State")
        w183 = u16 0 items=["Init array", "Send get", "recive data", "Close"] ("State")
        w192 = u16 0 items=["Init", "Write", "Read", "Close"] ("State")
        w197 = u8 23 items=["subscribe"=22, "startNetwork"=45, "setUser"=58, "setTime"=54, "setNetworkConfig"=26, "setLicense"=56, "setIPConfig"=68, "setDownstreamFrameMode"=51, "setCommonJoinKey"=66, "setAdvertising"=50, "setACLEntry"=39, "sendIP"=59, "sendData"=44, "restorFactoryDefaults"=61, "reset"=21, "radiotestTx"=35, "radiotestRx"=37, "pingMote"=42, "getTime"=23, "getSystemInfo"=46, "radiotestStatistics"=38, "getPathInfo"=48, "getNextPath"=49, "getNextACLEntry"=40, "getNetworkInfo"=64, "getNetworkConfig"=63, "getMoteLinks"=70, "getMoteInfo"=62, "getMoteConfigByld"=65, "getMoteConfig"=47, "getManagerStatistics"=53, "getLog"=43, "getLicense"=55, "getIPConfig"=67, "exchangeNetworkID"=34, "exchangeMoteJoinKey"=33, "deleteMote"=69, "deleteACLEntry"=41, "clearStatistics"=31] ("commandType_write")
        w198 = u16 1 items=["Connect", "Write", "Read", "Close"] ("State")
        w200 = u8 22 items=["subscribe"=22, "startNetwork"=45, "setUser"=58, "setTime"=54, "setNetworkConfig"=26, "setLicense"=56, "setIPConfig"=68, "setDownstreamFrameMode"=51, "setCommonJoinKey"=66, "setAdvertising"=50, "setACLEntry"=39, "sendIP"=59, "sendData"=44, "restorFactoryDefaults"=61, "reset"=21, "radiotestTx"=35, "radiotestRx"=37, "pingMote"=42, "getTime"=23, "getSystemInfo"=46, "radiotestStatistics"=38, "getPathInfo"=48, "getNextPath"=49, "getNextACLEntry"=40, "getNetworkInfo"=64, "getNetworkConfig"=63, "getMoteLinks"=70, "getMoteInfo"=62, "getMoteConfigByld"=65, "getMoteConfig"=47, "getManagerStatistics"=53, "getLog"=43, "getLicense"=55, "getIPConfig"=67, "exchangeNetworkID"=34, "exchangeMoteJoinKey"=33, "deleteMote"=69, "deleteACLEntry"=41, "clearStatistics"=31] ("commandType_write")
        w201 = u16 1 items=["Connect", "Write", "Read", "Close"] ("State")
        w203 = u16 0 items=["Connect", "Write", "Read", "Close"] ("State")
        n74 = call "rmad skredstorrelser initfile.vi"("initfile"=w171, "error in (no error)"=w179) -> ("Trafikkontroll terskelverdier"=w178:T2, "Stredstørrelser terskelverdier"=w180:T3, "error out"=w181:errorcluster)  [unwired: 9 in, 2 out]
        "Stredstørrelser terskelverdier" <- w180
        "Trafikkontroll terskelverdier" <- w178
        n75 = call "rmad logger initfile.vi"("initfile"=w171, "error in (no error)"=w181) -> ("mesh_datadir"=→"mesh_datadir":string, "aux_datadir"=→"aux_datadir":string, "event_datadir"=→"event_datadir":string, "serial mux"=w174:T31, "RMAD signalys monitor enabled"=w175:bool, "ini file"=→"ini file":path, "vdv_datadir"=→"vdv_datadir":string, "num sensors"=w167:u32[], "gateway_snmp"=w177:bool, "auto_download"=→"auto_download_enabled":bool, "mac adresses"=w185:T32, "error out"=w188:errorcluster)  [unwired: 1 in, 1 out]
        "gateway IP" <- w174
        "gateway_snmp_enabled" <- w177
        "RMAD signalys monitor enabled" <- w175
        n76 = call "RMAD skredstorrelse.vi"("State"=w182, "Stredstørrelser terskelverdier"=w180) -> ()  [unwired: 9 in, 5 out]
        n77 = Unbundle By Name(w185) -> ("node names"=→"node names":string[])
        n78 = call "traffic control controller.vi"("State"=w192, "Trafikkontroll terskelverdier"=w178) -> ()  [unwired: 11 in, 3 out]
        n79 = Unbundle By Name(w185) -> ("dust mac"=→"mac adress":string[])
        n80 = call "smartmeshIP serial mux IO.vi"("State"=w203, "error in"=w188, "serial mux adress"=w174) -> ("error out"=w202:errorcluster)  [unwired: 3 in, 5 out]
        n81 = Unbundle By Name(w185) -> ("dust master mac"=→"dust manager mac adress":string)
        n82 = call "smartmeshIP serial mux IO.vi"("tx_commandType"=w200, "State"=w201, "error in"=w202) -> ("error out"=w199:errorcluster)  [unwired: 3 in, 5 out]
        n83 = Unbundle By Name(w185) -> ("dust mac"=w195:string[])
        n84 = call "smartmeshIP serial mux IO.vi"("tx_commandType"=w197, "State"=w198, "error in"=w199) -> ("error out"=w196:errorcluster)  [unwired: 3 in, 5 out]
        n85 = for {
          shift-right: [w219] -> w165
          shift-left: w196 -> [w220]
          tunnel: w195 -> [w218] mode=indexing
          w222 = u16 1 items=["Connect", "Write", "Read", "Close"] ("State")
          w221 = u8 47 items=["subscribe"=22, "startNetwork"=45, "setUser"=58, "setTime"=54, "setNetworkConfig"=26, "setLicense"=56, "setIPConfig"=68, "setDownstreamFrameMode"=51, "setCommonJoinKey"=66, "setAdvertising"=50, "setACLEntry"=39, "sendIP"=59, "sendData"=44, "restorFactoryDefaults"=61, "reset"=21, "radiotestTx"=35, "radiotestRx"=37, "pingMote"=42, "getTime"=23, "getSystemInfo"=46, "radiotestStatistics"=38, "getPathInfo"=48, "getNextPath"=49, "getNextACLEntry"=40, "getNetworkInfo"=64, "getNetworkConfig"=63, "getMoteLinks"=70, "getMoteInfo"=62, "getMoteConfigByld"=65, "getMoteConfig"=47, "getManagerStatistics"=53, "getLog"=43, "getLicense"=55, "getIPConfig"=67, "exchangeNetworkID"=34, "exchangeMoteJoinKey"=33, "deleteMote"=69, "deleteACLEntry"=41, "clearStatistics"=31] ("commandType_write")
          n86 = call "smartmeshIP serial mux IO.vi"("tx_commandType"=w221, "State"=w222, "error in"=w220, "MAC source"=w218) -> ("error out"=w219:errorcluster)  [unwired: 2 in, 5 out]
        }
        n87 = Unbundle By Name(w174) -> ("serial_mux IP"=w173:string)
        n88 = case shown="True" w177 {
          tunnel: w165 -> [w207 w217]
          tunnel: [w207 w215] -> w184
          tunnel: w173 -> [_ w212]
          frame False {
          }
          frame True {
            w209 = u16 0 items=["Get Status", "Get Info", "Get Uptime"] ("Ring")
            w216 = u16 1 items=["Get Status", "Get Info", "Get Uptime"] ("Ring")
            n89 = call "spectre status snmp .vi"("Ring"=w216, "error in (no error)"=w217, "IP Address"=w212) -> ("error out"=w211:errorcluster, "Gateway Info"=w214:T16)  [unwired: 5 in, 2 out]
            "Gateway Info" <- w214
            n90 = call "spectre status snmp .vi"("Ring"=w209, "error in (no error)"=w211) -> ("error out"=w210:errorcluster, "Gateway Status"=w208:T17)  [unwired: 6 in, 2 out]
            n91 = Unbundle By Name(w214) -> ("Name"=w213:string)
            n92 = local write "Gateway Status"(w208) -> ()
            n93 = property class="VI"(error in=w210, "Front Panel.Title"=w213) -> (error out=w215:errorcluster)  [unwired: 1 in, 1 out]
          }
        }
        n94 = call "RMAD to RegObs.vi"("State"=w169) -> ("error out"=w164:errorcluster, "regobs from inifile"=→"regobs from inifile":T1, "baseurl"=→"regObs baseurl":string)  [unwired: 5 in, 3 out]
        n95 = call "NGI get dataset secure.vi"("num sensor"=w167, "error in (no error)"=w184, "State"=w183) -> ("error out"=w163:errorcluster)  [unwired: 13 in, 3 out]
        n96 = local write "error regObs"(w164) -> ()
        n97 = case shown="True" w175 {
          tunnel: w173 -> [_ w206]
          frame False {
          }
          frame True {
            n98 = call "traffic control monitor.vi"("address"=w206) -> ("error out"=w204:errorcluster, "RMAD Signalys Monitor"=w205:T18)  [unwired: 7 in, 2 out]
            n99 = local write "RMAD Signalys Monitor"(w205) -> ()
            n100 = local write "error signalys"(w204) -> ()
          }
        }
        n101 = Get Date/Time In Seconds() -> (seconds since 1Jan1904=w187:timestamp)
      }
    }
    "radio IO" <- w7
  }
  n102 = call "smartmeshIP serial mux IO.vi"("State"=w3, "error in"=w2) -> ()  [unwired: 4 in, 6 out]
